vi "Reflect Along Line.vi"(1 "Line End in":refnum<class "Vector2.lvclass">, 2 "Line Start in":refnum<class "Vector2.lvclass">, 3 "Vector in":refnum<class "Vector2.lvclass">) -> (0 "Vector out":refnum<class "Vector2.lvclass">)   [LabVIEW 2022 SP3, in "Vector2.lvclass"]
uses:
  Vector2.lvclass
  Vector2.lvclass/Vector2.ctl
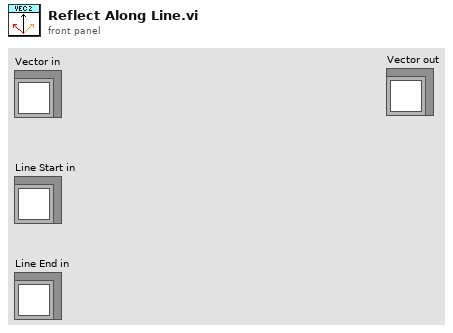
[diagram p1: front panel]
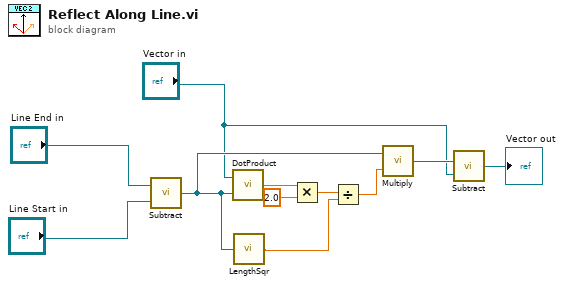
[diagram p0: block diagram]
diagram:
  n1 = call "Subtract.vi"("Vec2 b in"="Line Start in", "Vec2 a in"="Line End in") -> ("Vec2 out"=w4:refnum<class "Vector2.lvclass">)
  n2 = call "DotProduct.vi"("Vec2 b in"=w4, "Vec2 a in"="Vector in") -> ("Product out"=w9:sgl)
  n3 = call "LengthSqr.vi"("Vec2 in"=w4) -> ("Length Sqr out"=w6:sgl)
  n4 = Multiply(x=w9, y=sgl 2.0) -> (x*y=w7:sgl)
  n5 = Divide(x=w7, y=w6) -> (x/y=w5:sgl)
  n6 = call "Multiply.vi"("Scalar"=w5, "Vector in"=w4) -> ("Vector out"=w3:refnum<class "Vector2.lvclass">)
  n7 = call "Subtract.vi"("Vec2 b in"="Vector in", "Vec2 a in"=w3) -> ("Vec2 out"=→"Vector out":refnum<class "Vector2.lvclass">)
